vi "BRig_RT_panel_ExpStruct_v0,90.vi"(7 "input_setValues":bool, 11 "input_dataExp":u16[](array[numeric])) -> (3 "output_dataExp":u16[](array[numeric]))   [LabVIEW 2014]
panel:
  in  "FreeReward_Count2":u16
  in  "FreeReward_Count1":u16
  in  "FreeReward_Switch":bool
  in  "T_CuePenalty":u16=1000 caption="Penalty" min=1 max=10000 step=1
  in  "T_ENLPenalty":u16=100 caption="Penalty" min=10 max=10000 step=10
  in  "LaserSwitch_Probability_L1":u16
  in  "LaserSwitch":u16(slide) max=3 step=1 scale=0.0..3.0
  in  "I_allReward":bool caption="NonSpecific Lick Direction"
  in  "Tcycle_Reward_max_R":u16=1000 caption="Max" min=5 max=5000 step=5
  in  "Tcycle_Reward_min_R":u16=1000 caption="Min" min=5 max=5000 step=5
  in  "Tcycle_Reward_step_R":u16=1000 caption="Penalty" min=1 max=10000 step=1
  in  "Tcycle_Reward_max_L":u16=1000 caption="Max" min=5 max=5000 step=5
  in  "Tcycle_Reward_min_L":u16=1000 caption="Min" min=5 max=5000 step=5
  in  "Tcycle_Reward_step_L":u16=1000 caption="Penalty" min=1 max=10000 step=1
  in  "T_Cue_LED_max":u16=1000 caption="Max" min=5 max=5000 step=5
  in  "T_Cue_LED_min":u16=1000 caption="Min" min=5 max=5000 step=5
  in  "T_Cue_LED_step":u16=1000 caption="Penalty" min=1 max=10000 step=1
  in  "SolenoidProbability_L":u16=100 caption="Reward Time [ms]" min=1 max=1000 step=1
  in  "SolenoidProbability_R":u16=100 caption="Reward Time [ms]" min=1 max=1000 step=1
  in  "T_Cue_Audio_max":u16=1000 caption="Max" min=5 max=5000 step=5
  in  "T_Cue_Audio_min":u16=1000 caption="Min" min=5 max=5000 step=5
  in  "BUR_max":u16 caption="Count Reward Structure  (0 = off)"
  in  "Tcycle_Timeout":u16=1000 caption="Timeout Time [ms]" min=10 max=10000 step=1
  in  "Tcycle_Wrong":u16=1000 caption="Wrong Time [ms]" min=10 max=10000 step=1
  in  "Tcycle_Selection":u16=1000 caption="Answer Time [ms]" min=1 max=10000 step=1
  in  "Tcycle_RewardPost":u16=1000 caption="Consumption Time [ms]" min=250 max=10000 step=250
  in  "TpB_Max_R":u16=4 caption="Max TrialsPerBlock" min=1 max=12 step=1
  in  "TpB_Min_R":u16=4 caption="Min TrialsPerBlock" min=1 max=12 step=1
  in  "TpB_Max_L":u16=4 caption="Max TrialsPerBlock" min=1 max=12 step=1
  in  "TpB_Min_L":u16=4 caption="Min TrialsPerBlock" min=1 max=12 step=1
  in  "BUR_min":u16 caption="Count Reward Structure\n(0 = off)"
  in  "TrialUntilReward":bool caption="Ignore Wrong Selection"
  in  "T_Cue_Audio_step":u16=1000 caption="Penalty" min=1 max=10000 step=1
  in  "T_ENL_step":u16=100 caption="Penalty" min=10 max=10000 step=10
  in  "T_ENL_max":u16=1000 caption="Max" min=250 max=10000 step=250
  in  "T_ENL_min":u16=1000 caption="Min" min=250 max=10000 step=250
  # "Experiment Task Structure"
  # "Min            Max               Step        Penalty"
  # "Enforced\nNonLick"
  # "Cue Audio"
  # "Cue LED"
  # "Selection"
  # "Reward - Dispense Water"
  # "Min            Max            StepSize"
  # "Left"
  # "Right"
  # "Min"
  # "Max"
  # "Dispense Water Probability"
  # "%"
  # "Left"
  # "Trial Per Block Structure \n               Left                        Right"
  # "Right"
  # "%"
  # "Reward - Consumption"
  # "Min"
  # "Penalty - Wrong Choice"
  # "Max"
  # "Penalty - Choice Timeout"
  # "# consecutive ReBiasing trials"
  # "Give Reward\nIf Too Many Errors"
  # "# consecutive NonForcedError trials"
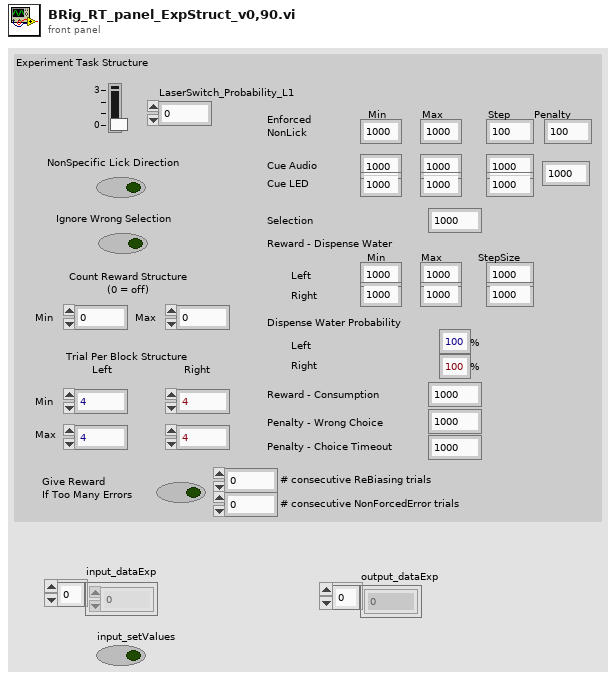
[diagram p1: front panel]
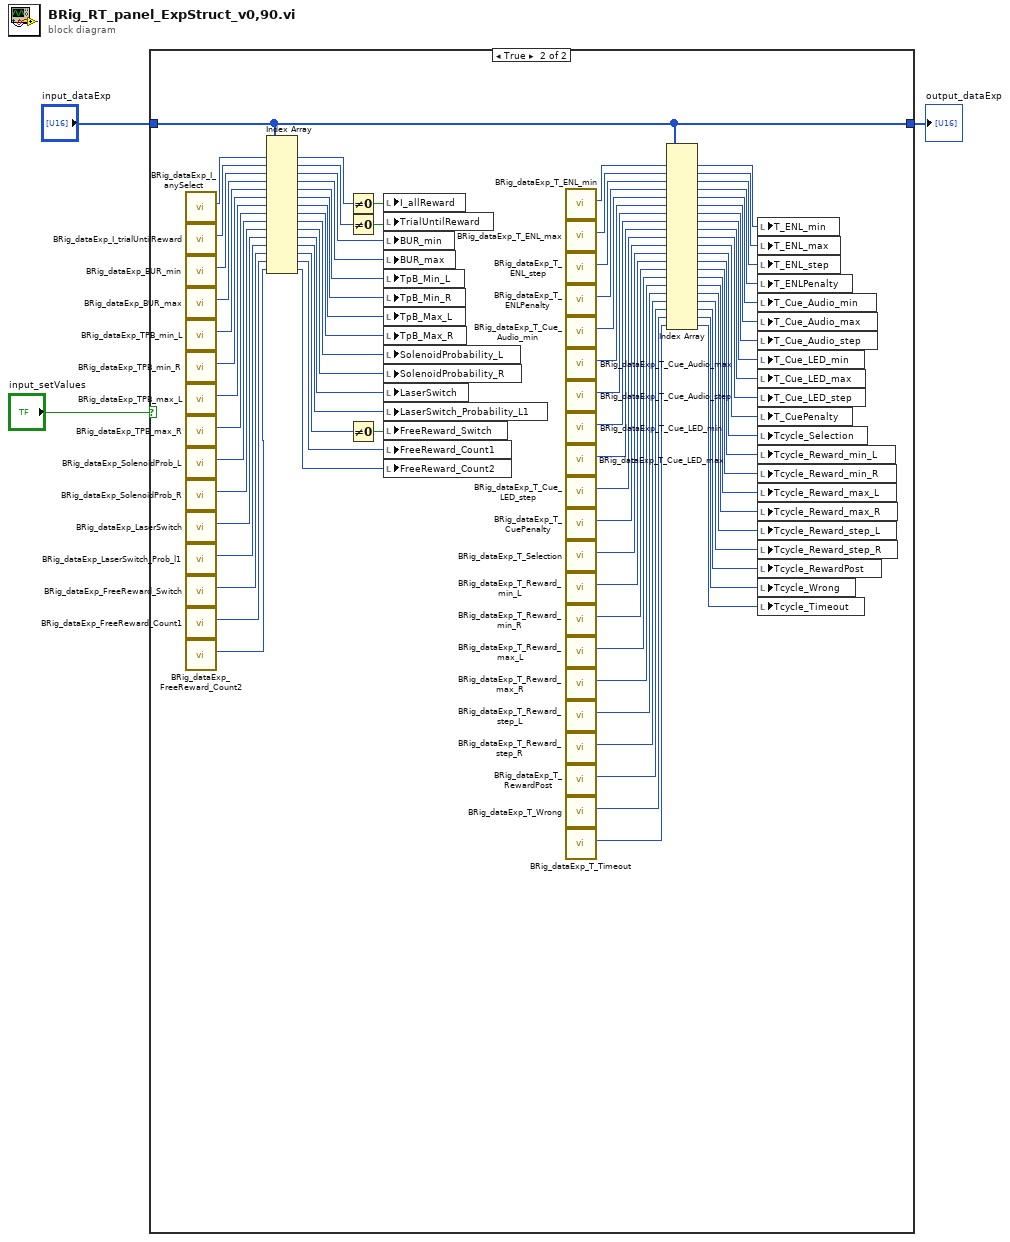
[diagram p0: block diagram]
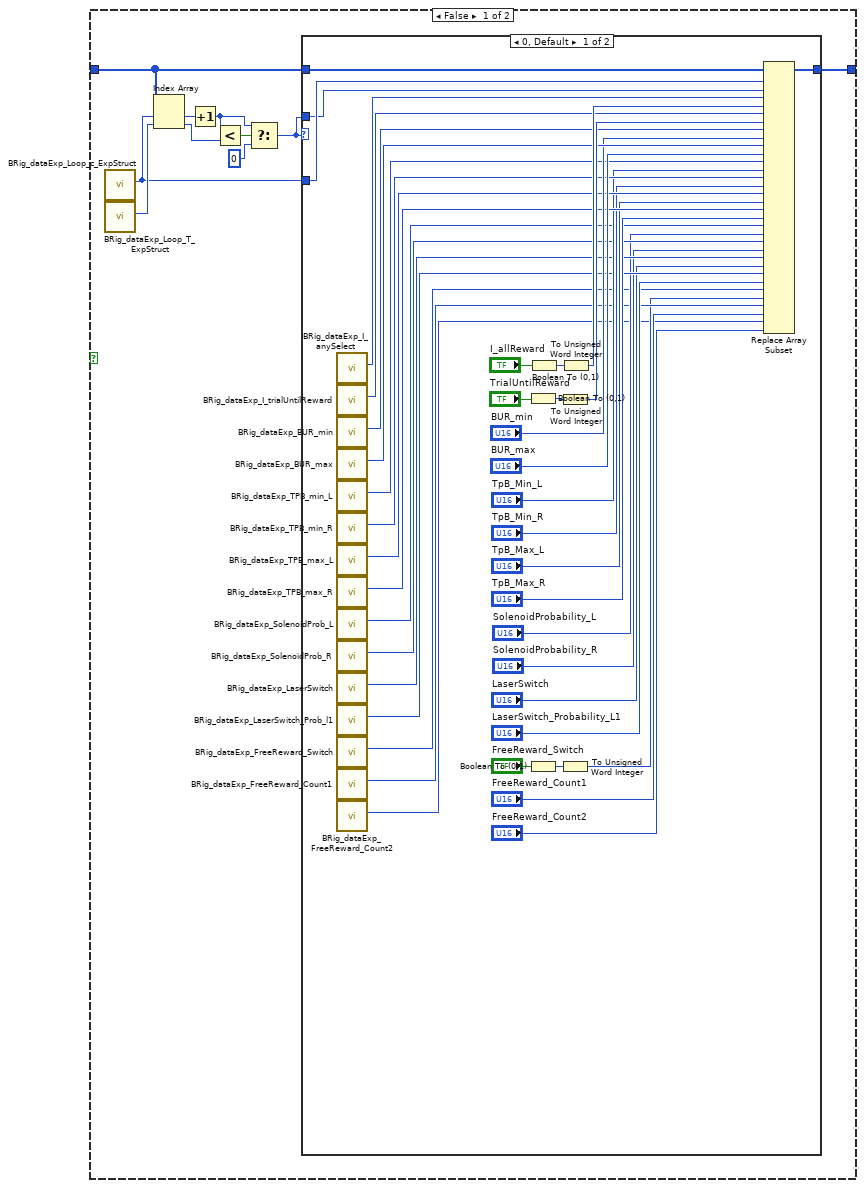
[diagram p2: hidden frame]
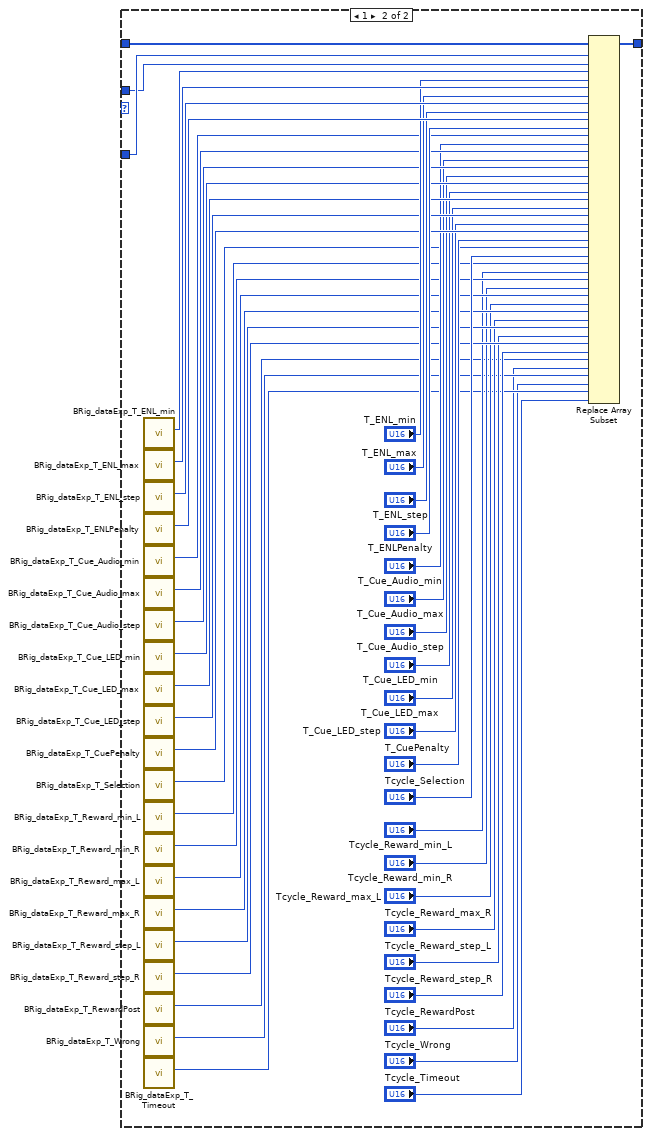
[diagram p3: hidden frame]
diagram:
  n1 = case shown="True" "input_setValues" {
    tunnel: [w13 w144] -> w3
    tunnel: "input_dataExp" -> [w12 w144]
    frame False {
      n2 = call "BRig_dataExp_Loop_c_ExpStruct.vi"() -> ("output_Loop_c_ExpStruct"=w6:i32)  [unwired: 11 in]
      n3 = call "BRig_dataExp_Loop_T_ExpStruct.vi"() -> ("output_Loop_T_ExpStruct"=w11:i32)  [unwired: 11 in]
      n4 = Index Array(array=w12, index #1=w6, index #2=w11) -> (element #1=w10:u16, element #2=w9:u16)
      n5 = Increment(x=w10) -> (x+1=w5:u16)
      n6 = Less?(x=w5, y=w9) -> (x < y?=w8:bool)
      n7 = Select(t=w5, s=w8, f=u16 0) -> (s? t:f=w4:u16)
      n8 = case shown="0, Default" w4 {
        tunnel: w12 -> [w53 w99]
        tunnel: [w52 w98] -> w13
        tunnel: w6 -> [w23 w97]
        tunnel: w4 -> [w22 w96]
        frame 0, Default {
          n9 = call "BRig_dataExp_I_anySelect.vi"() -> ("output_I_anySelect"=w51:i32)  [unwired: 11 in]
          n10 = call "BRig_dataExp_I_trialUntilReward.vi"() -> ("output_I_trialUntilReward"=w47:i32)  [unwired: 11 in]
          n11 = call "BRig_dataExp_BUR_min.vi"() -> ("output_BUR_min"=w43:i32)  [unwired: 11 in]
          n12 = call "BRig_dataExp_BUR_max.vi"() -> ("output_BUR_max"=w42:i32)  [unwired: 11 in]
          n13 = call "BRig_dataExp_TPB_min_L.vi"() -> ("output_TPB_min_L"=w39:i32)  [unwired: 11 in]
          n14 = call "BRig_dataExp_TPB_min_R.vi"() -> ("output_TPB_min_R"=w38:i32)  [unwired: 11 in]
          n15 = call "BRig_dataExp_TPB_max_L.vi"() -> ("output_TPB_max_L"=w37:i32)  [unwired: 11 in]
          n16 = call "BRig_dataExp_TPB_max_R.vi"() -> ("output_TPB_max_R"=w36:i32)  [unwired: 11 in]
          n17 = call "BRig_dataExp_SolenoidProb_L.vi"() -> ("output_SolenoidProbability_L"=w31:i32)  [unwired: 11 in]
          n18 = call "BRig_dataExp_SolenoidProb_R.vi"() -> ("output_SolenoidProbability_R"=w30:i32)  [unwired: 11 in]
          n19 = call "BRig_dataExp_LaserSwitch.vi"() -> ("output_LaserSwitch"=w29:i32)  [unwired: 11 in]
          n20 = call "BRig_dataExp_LaserSwitch_Prob_l1.vi"() -> ("output_LaserSwitch_Probability_L1"=w28:i32)  [unwired: 11 in]
          n21 = call "BRig_dataExp_FreeReward_Switch.vi"() -> ("output_FreeReward_Switch"=w19:i32)  [unwired: 11 in]
          n22 = call "BRig_dataExp_FreeReward_Count1.vi"() -> ("output_FreeReward_Count"=w18:i32)  [unwired: 11 in]
          n23 = call "BRig_dataExp_FreeReward_Count2.vi"() -> ("output_FreeReward_Count"=w15:i32)  [unwired: 11 in]
          n24 = Boolean To (0,1)(Boolean="TrialUntilReward") -> (0, 1=w46:i16)
          n25 = Boolean To (0,1)(Boolean="FreeReward_Switch") -> (0, 1=w21:i16)
          n26 = Boolean To (0,1)(Boolean="I_allReward") -> (0, 1=w49:i16)
          n27 = To Unsigned Word Integer(number=w46) -> (unsigned 16bit integer=w44:u16)
          n28 = To Unsigned Word Integer(number=w21) -> (unsigned 16bit integer=w17:u16)
          n29 = To Unsigned Word Integer(number=w49) -> (unsigned 16bit integer=w48:u16)
          n30 = Replace Array Subset(array=w53, new element #1=w22, index #1=w23, new element #2=w48, index #2=w51, new element #3=w44, index #3=w47, new element #4="BUR_min", index #4=w43, new element #5="BUR_max", index #5=w42, new element #6="TpB_Min_L", index #6=w39, new element #7="TpB_Min_R", index #7=w38, new element #8="TpB_Max_L", index #8=w37, new element #9="TpB_Max_R", index #9=w36, new element #10="SolenoidProbability_L", index #10=w31, new element #11="SolenoidProbability_R", index #11=w30, new element #12="LaserSwitch", index #12=w29, new element #13="LaserSwitch_Probability_L1", index #13=w28, new element #14=w17, index #14=w19, new element #15="FreeReward_Count1", index #15=w18, new element #16="FreeReward_Count2", index #16=w15) -> (w52:u16[])
        }
        frame 1 {
          n31 = call "BRig_dataExp_T_ENL_min.vi"() -> ("output_T_ENL_min"=w95:i32)  [unwired: 11 in]
          n32 = call "BRig_dataExp_T_ENL_max.vi"() -> ("output_T_ENL_max"=w94:i32)  [unwired: 11 in]
          n33 = call "BRig_dataExp_T_ENL_step.vi"() -> ("output_T_ENL_step"=w93:i32)  [unwired: 11 in]
          n34 = call "BRig_dataExp_T_ENLPenalty.vi"() -> ("output_ENL_penalty"=w92:i32)  [unwired: 11 in]
          n35 = call "BRig_dataExp_T_Cue_Audio_min.vi"() -> ("output_T_Cue_Audio_min"=w87:i32)  [unwired: 11 in]
          n36 = call "BRig_dataExp_T_Cue_Audio_max.vi"() -> ("output_T_Cue_Audio_max"=w86:i32)  [unwired: 11 in]
          n37 = call "BRig_dataExp_T_Cue_Audio_step.vi"() -> ("output_T_Cue_Audio_step"=w85:i32)  [unwired: 11 in]
          n38 = call "BRig_dataExp_T_Cue_LED_min.vi"() -> ("output_T_Cue_LED_min"=w84:i32)  [unwired: 11 in]
          n39 = call "BRig_dataExp_T_Cue_LED_max.vi"() -> ("output_T_Cue_LED_max"=w83:i32)  [unwired: 11 in]
          n40 = call "BRig_dataExp_T_Cue_LED_step.vi"() -> ("output_T_Cue_LED_step"=w82:i32)  [unwired: 11 in]
          n41 = call "BRig_dataExp_T_CuePenalty.vi"() -> ("output_T_CuePenalty"=w81:i32)  [unwired: 11 in]
          n42 = call "BRig_dataExp_T_Selection.vi"() -> ("output_T_Selection"=w73:i32)  [unwired: 11 in]
          n43 = call "BRig_dataExp_T_Reward_min_L.vi"() -> ("output_Tcycle_Reward_min_L"=w71:i32)  [unwired: 11 in]
          n44 = call "BRig_dataExp_T_Reward_min_R.vi"() -> ("output_T_Reward_min_R"=w70:i32)  [unwired: 11 in]
          n45 = call "BRig_dataExp_T_Reward_max_L.vi"() -> ("output_T_Reward_max_L"=w69:i32)  [unwired: 11 in]
          n46 = call "BRig_dataExp_T_Reward_max_R.vi"() -> ("output_T_Reward_max_R"=w68:i32)  [unwired: 11 in]
          n47 = call "BRig_dataExp_T_Reward_step_L.vi"() -> ("output_T_Reward_step_L"=w67:i32)  [unwired: 11 in]
          n48 = call "BRig_dataExp_T_Reward_step_R.vi"() -> ("output_T_Reward_step_R"=w66:i32)  [unwired: 11 in]
          n49 = call "BRig_dataExp_T_RewardPost.vi"() -> ("output_T_RewardPost"=w59:i32)  [unwired: 11 in]
          n50 = call "BRig_dataExp_T_Wrong.vi"() -> ("output_T_Wrong"=w58:i32)  [unwired: 11 in]
          n51 = call "BRig_dataExp_T_Timeout.vi"() -> ("output_T_Timeout"=w57:i32)  [unwired: 11 in]
          n52 = Replace Array Subset(array=w99, new element #1=w96, index #1=w97, new element #2="T_ENL_min", index #2=w95, new element #3="T_ENL_max", index #3=w94, new element #4="T_ENL_step", index #4=w93, new element #5="T_ENLPenalty", index #5=w92, new element #6="T_Cue_Audio_min", index #6=w87, new element #7="T_Cue_Audio_max", index #7=w86, new element #8="T_Cue_Audio_step", index #8=w85, new element #9="T_Cue_LED_min", index #9=w84, new element #10="T_Cue_LED_max", index #10=w83, new element #11="T_Cue_LED_step", index #11=w82, new element #12="T_CuePenalty", index #12=w81, new element #13="Tcycle_Selection", index #13=w73, new element #14="Tcycle_Reward_min_L", index #14=w71, new element #15="Tcycle_Reward_min_R", index #15=w70, new element #16="Tcycle_Reward_max_L", index #16=w69, new element #17="Tcycle_Reward_max_R", index #17=w68, new element #18="Tcycle_Reward_step_L", index #18=w67, new element #19="Tcycle_Reward_step_R", index #19=w66, new element #20="Tcycle_RewardPost", index #20=w59, new element #21="Tcycle_Wrong", index #21=w58, new element #22="Tcycle_Timeout", index #22=w57) -> (w98:u16[])
        }
      }
    }
    frame True {
      n53 = call "BRig_dataExp_I_anySelect.vi"() -> ("output_I_anySelect"=w175:i32)  [unwired: 11 in]
      n54 = call "BRig_dataExp_I_trialUntilReward.vi"() -> ("output_I_trialUntilReward"=w174:i32)  [unwired: 11 in]
      n55 = call "BRig_dataExp_BUR_min.vi"() -> ("output_BUR_min"=w173:i32)  [unwired: 11 in]
      n56 = call "BRig_dataExp_BUR_max.vi"() -> ("output_BUR_max"=w172:i32)  [unwired: 11 in]
      n57 = call "BRig_dataExp_TPB_min_L.vi"() -> ("output_TPB_min_L"=w171:i32)  [unwired: 11 in]
      n58 = call "BRig_dataExp_TPB_min_R.vi"() -> ("output_TPB_min_R"=w170:i32)  [unwired: 11 in]
      n59 = call "BRig_dataExp_TPB_max_L.vi"() -> ("output_TPB_max_L"=w169:i32)  [unwired: 11 in]
      n60 = call "BRig_dataExp_TPB_max_R.vi"() -> ("output_TPB_max_R"=w168:i32)  [unwired: 11 in]
      n61 = call "BRig_dataExp_SolenoidProb_L.vi"() -> ("output_SolenoidProbability_L"=w167:i32)  [unwired: 11 in]
      n62 = call "BRig_dataExp_SolenoidProb_R.vi"() -> ("output_SolenoidProbability_R"=w166:i32)  [unwired: 11 in]
      n63 = call "BRig_dataExp_LaserSwitch.vi"() -> ("output_LaserSwitch"=w165:i32)  [unwired: 11 in]
      n64 = call "BRig_dataExp_LaserSwitch_Prob_l1.vi"() -> ("output_LaserSwitch_Probability_L1"=w164:i32)  [unwired: 11 in]
      n65 = call "BRig_dataExp_FreeReward_Switch.vi"() -> ("output_FreeReward_Switch"=w163:i32)  [unwired: 11 in]
      n66 = call "BRig_dataExp_FreeReward_Count1.vi"() -> ("output_FreeReward_Count"=w162:i32)  [unwired: 11 in]
      n67 = call "BRig_dataExp_FreeReward_Count2.vi"() -> ("output_FreeReward_Count"=w101:i32)  [unwired: 11 in]
      n68 = Index Array(array=w144, index #1=w175, index #2=w174, index #3=w173, index #4=w172, index #5=w171, index #6=w170, index #7=w169, index #8=w168, index #9=w167, index #10=w166, index #11=w165, index #12=w164, index #13=w163, index #14=w162, index #15=w101) -> (element #1=w158:u16, element #2=w157:u16, element #3=w156:u16, element #4=w155:u16, element #5=w154:u16, element #6=w153:u16, element #7=w152:u16, element #8=w151:u16, element #9=w150:u16, element #10=w149:u16, element #11=w148:u16, element #12=w147:u16, element #13=w146:u16, element #14=w145:u16, element #15=w100:u16)
      n69 = Not Equal To 0?(x=w158) -> (x != 0?=w161:bool)
      n70 = Not Equal To 0?(x=w157) -> (x != 0?=w160:bool)
      n71 = Not Equal To 0?(x=w146) -> (x != 0?=w159:bool)
      n72 = local write "I_allReward"(w161) -> ()
      n73 = local write "TrialUntilReward"(w160) -> ()
      n74 = local write "BUR_min"(w156) -> ()
      n75 = local write "BUR_max"(w155) -> ()
      n76 = local write "TpB_Min_L"(w154) -> ()
      n77 = local write "TpB_Min_R"(w153) -> ()
      n78 = local write "TpB_Max_L"(w152) -> ()
      n79 = local write "TpB_Max_R"(w151) -> ()
      n80 = local write "SolenoidProbability_L"(w150) -> ()
      n81 = local write "SolenoidProbability_R"(w149) -> ()
      n82 = local write "LaserSwitch"(w148) -> ()
      n83 = local write "LaserSwitch_Probability_L1"(w147) -> ()
      n84 = local write "FreeReward_Switch"(w159) -> ()
      n85 = local write "FreeReward_Count1"(w145) -> ()
      n86 = local write "FreeReward_Count2"(w100) -> ()
      n87 = call "BRig_dataExp_T_ENL_min.vi"() -> ("output_T_ENL_min"=w143:i32)  [unwired: 11 in]
      n88 = call "BRig_dataExp_T_ENL_max.vi"() -> ("output_T_ENL_max"=w142:i32)  [unwired: 11 in]
      n89 = call "BRig_dataExp_T_ENL_step.vi"() -> ("output_T_ENL_step"=w141:i32)  [unwired: 11 in]
      n90 = call "BRig_dataExp_T_ENLPenalty.vi"() -> ("output_ENL_penalty"=w140:i32)  [unwired: 11 in]
      n91 = call "BRig_dataExp_T_Cue_Audio_min.vi"() -> ("output_T_Cue_Audio_min"=w139:i32)  [unwired: 11 in]
      n92 = call "BRig_dataExp_T_Cue_Audio_max.vi"() -> ("output_T_Cue_Audio_max"=w138:i32)  [unwired: 11 in]
      n93 = call "BRig_dataExp_T_Cue_Audio_step.vi"() -> ("output_T_Cue_Audio_step"=w137:i32)  [unwired: 11 in]
      n94 = call "BRig_dataExp_T_Cue_LED_min.vi"() -> ("output_T_Cue_LED_min"=w136:i32)  [unwired: 11 in]
      n95 = call "BRig_dataExp_T_Cue_LED_max.vi"() -> ("output_T_Cue_LED_max"=w135:i32)  [unwired: 11 in]
      n96 = call "BRig_dataExp_T_Cue_LED_step.vi"() -> ("output_T_Cue_LED_step"=w134:i32)  [unwired: 11 in]
      n97 = call "BRig_dataExp_T_CuePenalty.vi"() -> ("output_T_CuePenalty"=w133:i32)  [unwired: 11 in]
      n98 = call "BRig_dataExp_T_Selection.vi"() -> ("output_T_Selection"=w132:i32)  [unwired: 11 in]
      n99 = call "BRig_dataExp_T_Reward_min_L.vi"() -> ("output_Tcycle_Reward_min_L"=w131:i32)  [unwired: 11 in]
      n100 = call "BRig_dataExp_T_Reward_min_R.vi"() -> ("output_T_Reward_min_R"=w130:i32)  [unwired: 11 in]
      n101 = call "BRig_dataExp_T_Reward_max_L.vi"() -> ("output_T_Reward_max_L"=w129:i32)  [unwired: 11 in]
      n102 = call "BRig_dataExp_T_Reward_max_R.vi"() -> ("output_T_Reward_max_R"=w128:i32)  [unwired: 11 in]
      n103 = call "BRig_dataExp_T_Reward_step_L.vi"() -> ("output_T_Reward_step_L"=w127:i32)  [unwired: 11 in]
      n104 = call "BRig_dataExp_T_Reward_step_R.vi"() -> ("output_T_Reward_step_R"=w126:i32)  [unwired: 11 in]
      n105 = call "BRig_dataExp_T_RewardPost.vi"() -> ("output_T_RewardPost"=w125:i32)  [unwired: 11 in]
      n106 = call "BRig_dataExp_T_Wrong.vi"() -> ("output_T_Wrong"=w124:i32)  [unwired: 11 in]
      n107 = call "BRig_dataExp_T_Timeout.vi"() -> ("output_T_Timeout"=w123:i32)  [unwired: 11 in]
      n108 = Index Array(array=w144, index #1=w143, index #2=w142, index #3=w141, index #4=w140, index #5=w139, index #6=w138, index #7=w137, index #8=w136, index #9=w135, index #10=w134, index #11=w133, index #12=w132, index #13=w131, index #14=w130, index #15=w129, index #16=w128, index #17=w127, index #18=w126, index #19=w125, index #20=w124, index #21=w123) -> (element #1=w122:u16, element #2=w121:u16, element #3=w120:u16, element #4=w119:u16, element #5=w118:u16, element #6=w117:u16, element #7=w116:u16, element #8=w115:u16, element #9=w114:u16, element #10=w113:u16, element #11=w112:u16, element #12=w111:u16, element #13=w110:u16, element #14=w109:u16, element #15=w108:u16, element #16=w107:u16, element #17=w106:u16, element #18=w105:u16, element #19=w104:u16, element #20=w103:u16, element #21=w102:u16)
      n109 = local write "T_ENL_min"(w122) -> ()
      n110 = local write "T_ENL_max"(w121) -> ()
      n111 = local write "T_ENL_step"(w120) -> ()
      n112 = local write "T_ENLPenalty"(w119) -> ()
      n113 = local write "T_Cue_Audio_min"(w118) -> ()
      n114 = local write "T_Cue_Audio_max"(w117) -> ()
      n115 = local write "T_Cue_Audio_step"(w116) -> ()
      n116 = local write "T_Cue_LED_min"(w115) -> ()
      n117 = local write "T_Cue_LED_max"(w114) -> ()
      n118 = local write "T_Cue_LED_step"(w113) -> ()
      n119 = local write "T_CuePenalty"(w112) -> ()
      n120 = local write "Tcycle_Selection"(w111) -> ()
      n121 = local write "Tcycle_Reward_min_L"(w110) -> ()
      n122 = local write "Tcycle_Reward_min_R"(w109) -> ()
      n123 = local write "Tcycle_Reward_max_L"(w108) -> ()
      n124 = local write "Tcycle_Reward_max_R"(w107) -> ()
      n125 = local write "Tcycle_Reward_step_L"(w106) -> ()
      n126 = local write "Tcycle_Reward_step_R"(w105) -> ()
      n127 = local write "Tcycle_RewardPost"(w104) -> ()
      n128 = local write "Tcycle_Wrong"(w103) -> ()
      n129 = local write "Tcycle_Timeout"(w102) -> ()
    }
  }
  "output_dataExp" <- w3
